vi "Platform_initialization.vi"(8 "error in (no error)":errorcluster, 11 "Modeli in":refnum<class "Modeli.lvclass">) -> (0 "error out":errorcluster, 3 "Modeli out":refnum<class "Modeli.lvclass">)   [LabVIEW 2018, in "Modeli.lvlib" / "Modeli.lvclass"]
uses:
  Modeli.lvclass
  Projects/PRJ-Quasar Listening/Quasar Listening/x64/Release/Quasar Listening.dll
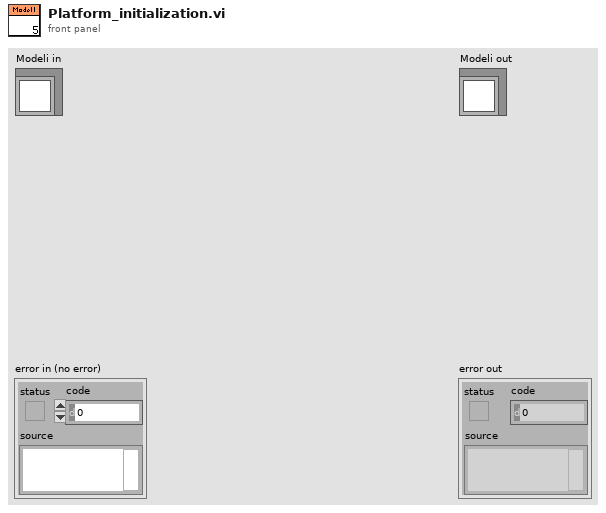
[diagram p1: front panel]
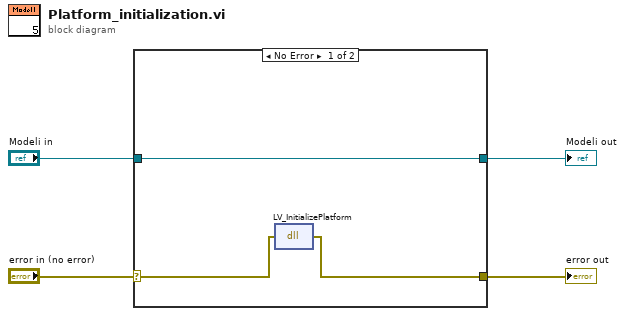
[diagram p0: block diagram]
diagram:
  n1 = case shown="No Error" "error in (no error)" {
    selector: "error in (no error)" -> [w6 w9]
    tunnel: [w5 w9] -> w3
    tunnel: [w7 w8] -> w1
    tunnel: "Modeli in" -> [w7 w8]
    frame No Error {
      n2 = dll-call lib="C:/Projects/PRJ-Quasar Listening/Quasar Listening/x64/Release/Quasar Listening.dll" fn="LV_InitializePlatform"(error in=w6) -> (error out=w5:errorcluster)  [unwired: 3 in, 1 out]
    }
    frame Error {
    }
  }
  "error out" <- w3
  "Modeli out" <- w1
